vi "GPSGGA.vi"(0 "String":string) -> (1 "Altitud":string, 2 "Sep Geoide":string, 3 "Ubicación":string, 4 "Hora":string, 5 "Fix Status":string, 6 "# Satelite":string)   [LabVIEW 2020]
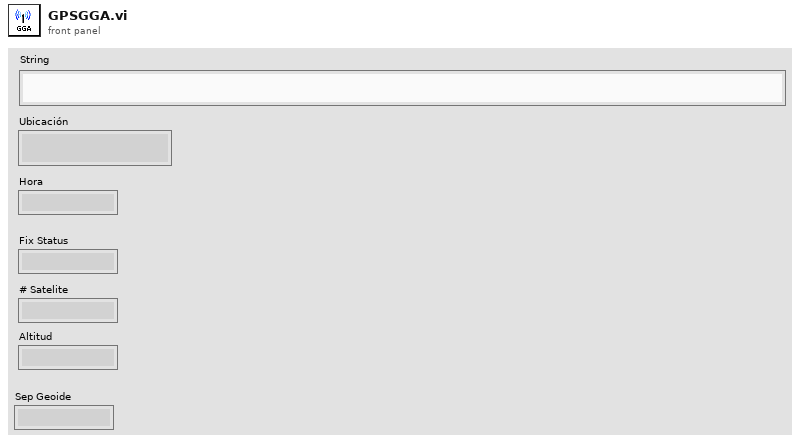
[diagram p1: front panel]
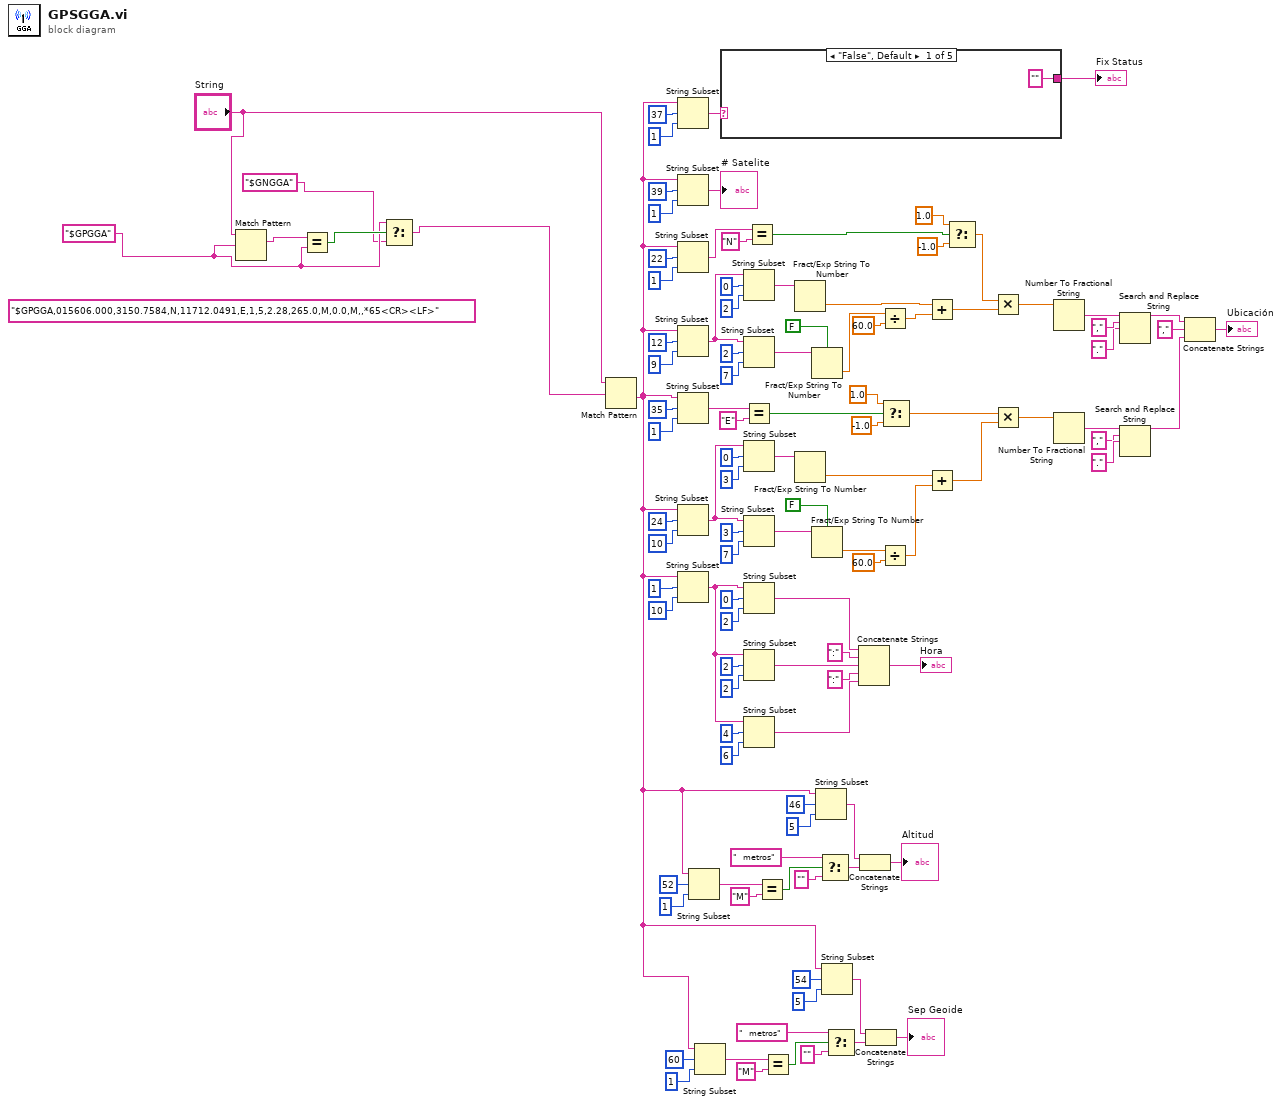
[diagram p0: block diagram]
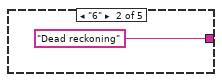
[diagram p2: hidden frame]
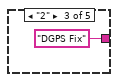
[diagram p3: hidden frame]
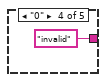
[diagram p4: hidden frame]
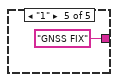
[diagram p5: hidden frame]
diagram:
  w3 = "$GPGGA" ("regular expression")
  (unwired) "$GPGGA,015606.000,3150.7584,N,11712.0491,E,1,5,2.28,265.0,M,0.0,M,,*65<CR><LF>"
  n1 = Match Pattern(string="String", regular expression=w3) -> (match substring=w6:string)  [unwired: 1 in, 3 out]
  n2 = Equal?(x=w6, y=w3) -> (x = y?=w5:bool)
  n3 = Select(t=w3, s=w5, f="$GNGGA" ("regular expression")) -> (s? t:f=w4:string)
  n4 = Match Pattern(string="String", regular expression=w4) -> (after substring=w7:string)  [unwired: 1 in, 3 out]
  n5 = String Subset(string=w7, offset (0)=37, length (rest)=1 ("length (rest)")) -> (substring=w33:string)
  n6 = String Subset(string=w7, offset (0)=39, length (rest)=1 ("length (rest)")) -> (substring=→"# Satelite":string)
  n7 = String Subset(string=w7, offset (0)=22, length (rest)=1 ("length (rest)")) -> (substring=w93:string)
  n8 = String Subset(string=w7, offset (0)=12, length (rest)=9 ("length (rest)")) -> (substring=w105:string)
  n9 = String Subset(string=w7, offset (0)=35, length (rest)=1 ("length (rest)")) -> (substring=w67:string)
  n10 = String Subset(string=w7, offset (0)=24, length (rest)=10 ("length (rest)")) -> (substring=w77:string)
  n11 = String Subset(string=w7, offset (0)=1, length (rest)=10 ("length (rest)")) -> (substring=w48:string)
  n12 = String Subset(string=w7, offset (0)=52, length (rest)=1 ("length (rest)")) -> (substring=w26:string)
  n13 = String Subset(string=w7, offset (0)=60, length (rest)=1 ("length (rest)")) -> (substring=w13:string)
  n14 = case shown="\"False\", Default" w33 {
    tunnel: ["" "Dead reckoning" "DGPS Fix" "invalid" "GNSS FIX"] -> w32
    frame "False", Default {
    }
    frame "6" {
    }
    frame "2" {
    }
    frame "0" {
    }
    frame "1" {
    }
  }
  "Fix Status" <- w32
  n15 = String Subset(string=w105, offset (0)=0, length (rest)=2 ("length (rest)")) -> (substring=w101:string)
  n16 = String Subset(string=w105, offset (0)=2, length (rest)=7 ("length (rest)")) -> (substring=w102:string)
  n17 = Equal?(x=w67, y="E") -> (x = y?=w69:bool)
  n18 = String Subset(string=w77, offset (0)=0, length (rest)=3 ("length (rest)")) -> (substring=w81:string)
  n19 = String Subset(string=w77, offset (0)=3, length (rest)=7 ("length (rest)")) -> (substring=w80:string)
  n20 = String Subset(string=w48, offset (0)=0, length (rest)=2 ("length (rest)")) -> (substring=w45:string)
  n21 = String Subset(string=w48, offset (0)=2, length (rest)=2 ("length (rest)")) -> (substring=w43:string)
  n22 = String Subset(string=w48, offset (0)=4, length (rest)=6 ("length (rest)")) -> (substring=w41:string)
  n23 = Equal?(x=w93, y="N") -> (x = y?=w91:bool)
  n24 = Equal?(x=w26, y="M") -> (x = y?=w24:bool)
  n25 = Equal?(x=w13, y="M") -> (x = y?=w15:bool)
  n26 = Fract/Exp String To Number(string=w101) -> (number=w97:dbl)  [unwired: 3 in, 1 out]
  n27 = Fract/Exp String To Number(string=w81) -> (number=w85:dbl)  [unwired: 3 in, 1 out]
  n28 = Fract/Exp String To Number(use system decimal point (T)=FALSE, string=w102) -> (number=w99:dbl)  [unwired: 2 in, 1 out]
  n29 = Fract/Exp String To Number(use system decimal point (T)=FALSE, string=w80) -> (number=w83:dbl)  [unwired: 2 in, 1 out]
  n30 = String Subset(string=w7, offset (0)=46, length (rest)=5 ("length (rest)")) -> (substring=w27:string)
  n31 = Select(t="  metros", s=w24, f="") -> (s? t:f=w21:string)
  n32 = String Subset(string=w7, offset (0)=54, length (rest)=5 ("length (rest)")) -> (substring=w12:string)
  n33 = Select(t="  metros", s=w15, f="") -> (s? t:f=w18:string)
  n34 = Concatenate Strings(w45, ":" ("string"), w43, ":" ("string"), w41) -> (→"Hora":string)
  n35 = Concatenate Strings(w27, w21) -> (→"Altitud":string)
  n36 = Concatenate Strings(w12, w18) -> (→"Sep Geoide":string)
  n37 = Divide(x=w99, y=60.0) -> (x/y=w96:dbl)
  n38 = Divide(x=w83, y=60.0) -> (x/y=w86:dbl)
  n39 = Select(t=1.0, s=w69, f=-1.0) -> (s? t:f=w72:dbl)
  n40 = Add(x=w97, y=w96) -> (x+y=w87:dbl)
  n41 = Add(x=w85, y=w86) -> (x+y=w66:dbl)
  n42 = Select(t=1.0, s=w91, f=-1.0) -> (s? t:f=w88:dbl)
  n43 = Multiply(x=w88, y=w87) -> (x*y=w63:dbl)
  n44 = Multiply(x=w72, y=w66) -> (x*y=w62:dbl)
  n45 = Number To Fractional String(number=w63) -> (F-format string=w61:string)  [unwired: 3 in]
  n46 = Number To Fractional String(number=w62) -> (F-format string=w56:string)  [unwired: 3 in]
  n47 = Search and Replace String(input string=w61, search string=",", replace string="." ("replace string (\"\")")) -> (result string=w53:string)  [unwired: 5 in, 3 out]
  n48 = Search and Replace String(input string=w56, search string=",", replace string="." ("replace string (\"\")")) -> (result string=w55:string)  [unwired: 5 in, 3 out]
  n49 = Concatenate Strings(w53, "," ("string"), w55) -> (→"Ubicación":string)
